vi "TruncI32.vi"(5 "Decimal places":i8, 6 "Number":i32) -> (2 "Truncated number":i32)   [LabVIEW 2017, in "GPNumeric.lvlib"]
doc: "Truncates <B>Number</B> to a number of <B>Decimal places</B>.\n\nSet <B>Decimal places</B> to a negative number to truncate to nearest 10, nearest 100 and so on. E.g. to truncate 782 to the nearest hundred, you set <B>Decimal places</B> to -2 and the <B>Truncated number</B> will be 700.\n\nThis VI is inlined.\n\nSteen Schmidt\nGPower\n16/5 2014"
uses:
  GPNumeric.lvlib
panel:
  # "Copyright © 2014\nGPower\nSee enclosed license file for terms and conditions"
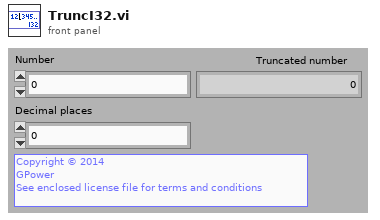
[diagram p1: front panel]
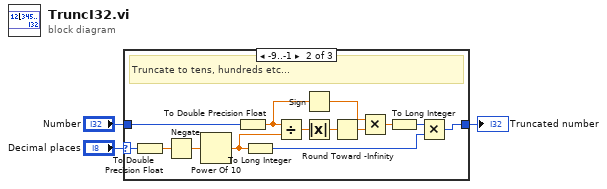
[diagram p0: block diagram]
diagram:
  n1 = case shown="-9..-1" "Decimal places" {
    selector: "Decimal places" -> [_ w14 _]
    tunnel: [_ w11 w18] -> w3
    tunnel: "Number" -> [_ w12 w18]
    frame ..-10 {
      # "Truncate above max value; Return zero."
    }
    frame -9..-1 {
      # "Truncate to tens, hundreds etc..."
      n2 = To Double Precision Float(number=w14) -> (double precision float=w13:dbl)
      n3 = Negate(x=w13) -> (-x=w17:dbl)
      n4 = Power Of 10(x=w17) -> (10^x=w10:dbl)
      n5 = To Double Precision Float(number=w12) -> (double precision float=w5:dbl)
      n6 = To Long Integer(number=w10) -> (32bit integer=w16:i32)
      n7 = Divide(x=w5, y=w10) -> (x/y=w4:dbl)
      n8 = Sign(1:w5) -> (0:w6:dbl)
      n9 = Absolute Value(x=w4) -> (abs(x)=w9:dbl)
      n10 = Round Toward -Infinity(1:w9) -> (0:w8:dbl)
      n11 = Multiply(x=w6, y=w8) -> (x*y=w7:dbl)
      n12 = To Long Integer(number=w7) -> (32bit integer=w15:i32)
      n13 = Multiply(x=w15, y=w16) -> (x*y=w11:i32)
    }
    frame 0.. {
      # "Truncate to n decimal places; return integer unchanged."
    }
  }
  "Truncated number" <- w3
